vi "归一化优化算法.vi"(9 "光源散斑簇":T2, 10 "散斑图像作用结果（处理）":dbl[](array[numeric]), 11 "模块选择簇":T1) -> (3 "归一化优化重建图像重排一维数组":dbl[](array[numeric]))   [LabVIEW 2018]
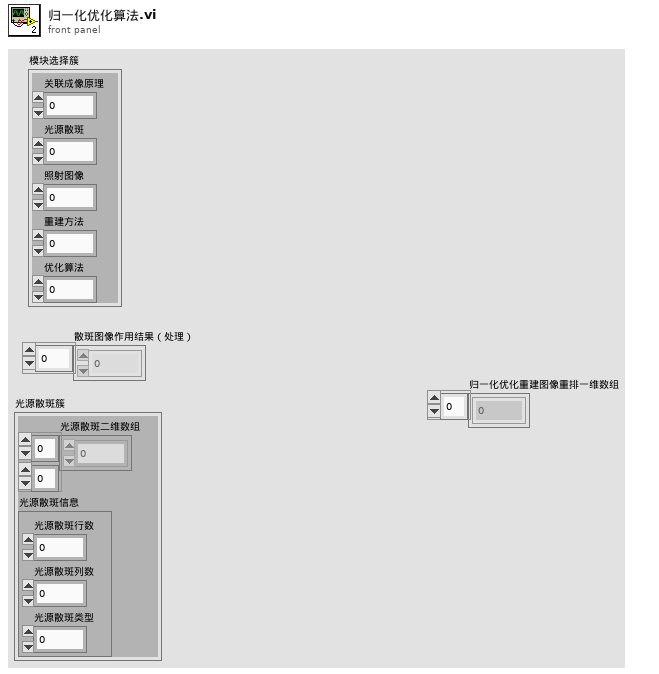
[diagram p1: front panel]
types:
  T1 = cluster{"关联成像原理":i32, "光源散斑":i32, "照射图像":i32, "重建方法":i32, "优化算法":i32}
  T2 = cluster{"光源散斑二维数组":dbl[][], "光源散斑信息":cluster{"光源散斑行数":dbl, "光源散斑列数":dbl, "光源散斑类型":dbl}}
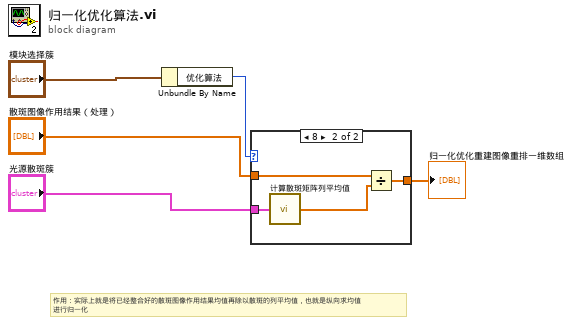
[diagram p0: block diagram]
diagram:
  # "作用：实际上就是将已经整合好的散斑图像作用结果均值再除以散斑的列平均值，也就是纵向求均值\n进行归一化"
  n1 = Unbundle By Name("模块选择簇") -> ("优化算法"=w4:i32)
  n2 = case shown="8" w4 {
    tunnel: "散斑图像作用结果（处理）" -> [w6 w9]
    tunnel: "光源散斑簇" -> [_ w8]
    tunnel: [w6 w7] -> w1
    frame 0, Default {
    }
    frame 8 {
      n3 = call "计算散斑矩阵列平均值.vi"("光源散斑簇"=w8) -> ("散斑二维数组列平均值"=w10:dbl[])
      n4 = Divide(x=w9, y=w10) -> (x/y=w7:dbl[])
    }
  }
  "归一化优化重建图像重排一维数组" <- w1
